vi "REACTOR__SET_REPETICIONES.vi"(6 "error in (no error)":errorcluster, 7 "Index":i8) -> (0 "error out":errorcluster, 1 "resulting string 2":string="Mide Bronkhorst 1, mide Alicats 1,  y pausa 1.0s", 2 "resulting string 1":string="Mide Bronkhorst 1, mide Alicats 1,  y pausa 1.0s", 3 "Cancelled?":bool)   [LabVIEW 2017]
doc: "Use this template to create a dialog box. This template polls the state of the buttons on the front panel and does not use events. Use the Dialog Using Events template (not available in Base package) to create a dialog box with event handling."
panel:
  in  "#REPETICIONES":i32=5
  in  "Cancel":bool
  in  "OK":bool
  # "REPETICIONES"
  # "Coloque los comandos a repetir\nentre las líneas de inicio y fin de \nrepeticiones"
  # "Noviembre 2022 V1.0  a-sslcdms"
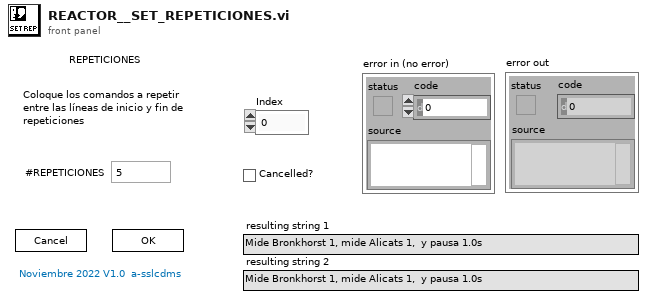
[diagram p1: front panel]
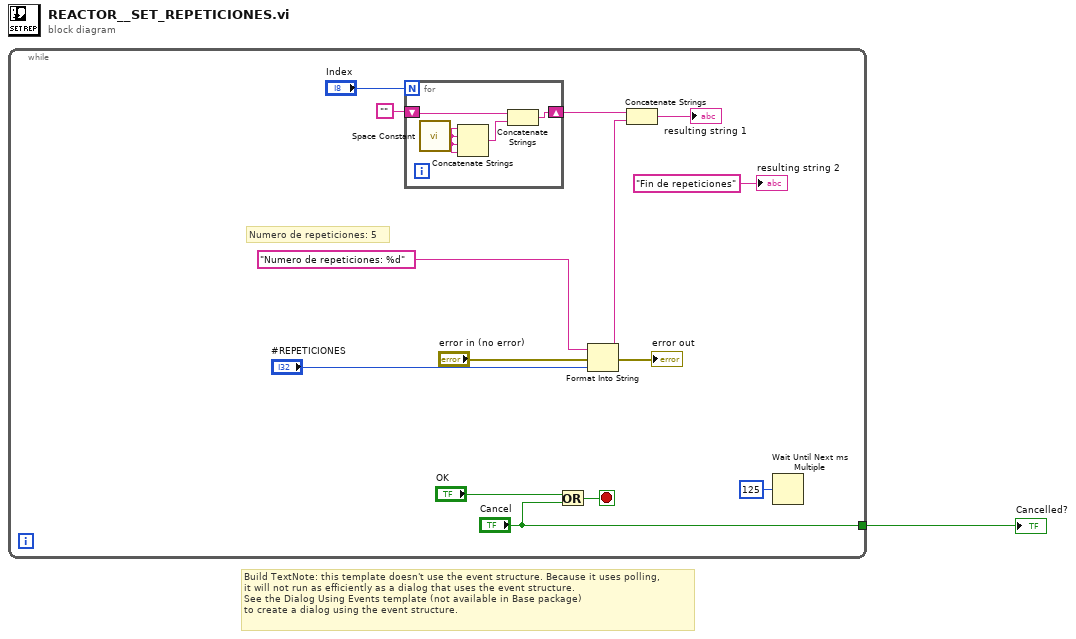
[diagram p0: block diagram]
diagram:
  # "Build TextNote: this template doesn't use the event structure. Because it uses polling, \nit will not run as efficiently as a dialog that uses the event structure.\nSee the Dialog Using Events template (not available in Base package) \nto create a dialog using the event structure."
  n1 = while {
    tunnel: ["Cancel"] -> w1
    stop <- w14 stop-if-true
    # "Numero de repeticiones: 5"
    n2 = for {
      N: "Index" -> [_]
      shift-right: [w18] -> w6
      shift-left: "" -> [w17]
      n3 = call <vilib>:"Space Constant.vi"() -> ("String"=w16:string)
      n4 = Concatenate Strings(w16, w16, w16, w16) -> (w19:string)
      n5 = Concatenate Strings(w17, w19) -> (w18:string)
    }
    n6 = Or(x="OK", y="Cancel") -> (x .or. y?=w14:bool)
    n7 = Format Into String(format string="Numero de repeticiones: %d", error in="error in (no error)", "#REPETICIONES") -> (resulting string=w4:string, error out=→"error out":errorcluster)  [unwired: 1 in]
    n8 = Concatenate Strings(w6, w4) -> (→"resulting string 1":string)
    n9 = Wait Until Next ms Multiple(millisecond multiple=u32 125) -> ()  [unwired: 1 out]
    "resulting string 2" <- "Fin de repeticiones" ("format string")
  }
  "Cancelled?" <- w1
